vi "Throughput Test.vi"() -> ()   [LabVIEW 2017]
uses:
  logger/Logger.lvclass
panel:
  out "error IO":errorcluster
  out "tag count":i32
  out "Running":bool
  out "tag updates":i32
  out "tag publish interval":i32
  out "Iteration":i32
  in  "stop":bool
  in  "File Send Interval (Seconds)":dbl=600.0
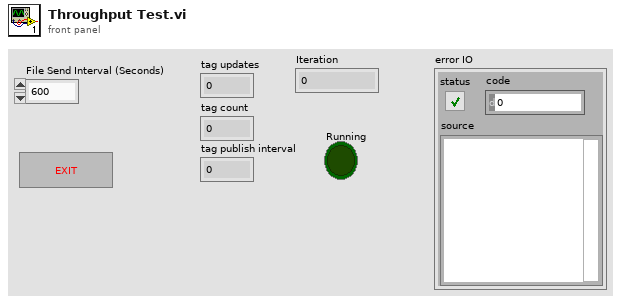
[diagram p1: front panel]
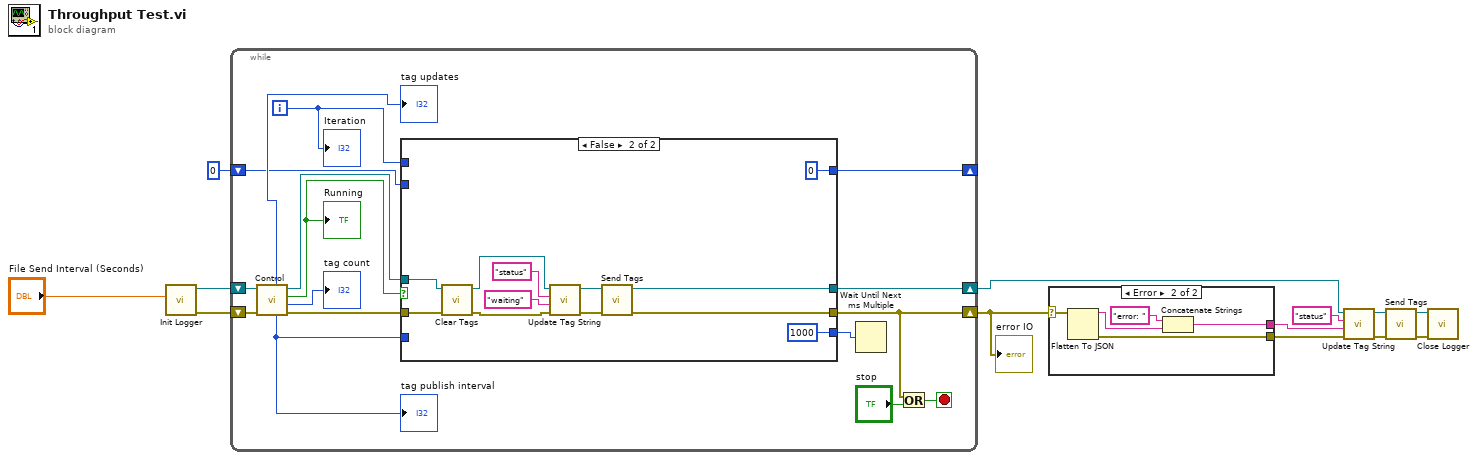
[diagram p0: block diagram]
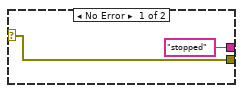
[diagram p2: hidden frame]
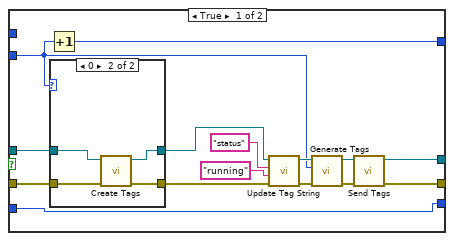
[diagram p3: hidden frame]
diagram:
  n1 = call "Init Logger.vi"("File Send Interval (Seconds)"="File Send Interval (Seconds)") -> ("error out"=w11:errorcluster, "Logger out.lvclass"=w12:refnum<class "Logger.lvclass">)  [unwired: 9 in]
  n2 = while {
    shift-right: [w24] -> w2
    shift-left: w11 -> [w19]
    shift-right: [w26] -> w6
    shift-left: w12 -> [w20]
    shift-right: [w14] -> _
    shift-left: 0 -> [w15]
    i -> [w16]
    stop <- w23 stop-if-true
    n3 = call "Control.vi"("error in (no error)"=w19, "Logger in.lvclass"=w20) -> ("error out"=w28:errorcluster, "tag count"=→"tag count":i32, "Start"=w29:bool, "Logger out.lvclass"=w27:refnum<class "Logger.lvclass">, "tag publish interval"=w18:i32, "tag updates"=→"tag updates":i32)  [unwired: 4 in]
    "tag publish interval" <- w18
    "Running" <- w29
    n4 = case shown="False" w29 {
      tunnel: w28 -> [w32 w57]
      tunnel: [w44 w62] -> w24
      tunnel: w27 -> [w30 w58]
      tunnel: [w43 w61] -> w26
      tunnel: w18 -> [w36 _]
      tunnel: [w36 1000 ("tag publish interval")] -> w17
      tunnel: w16 -> [_ _]
      tunnel: w15 -> [w34 _]
      tunnel: [w35 0] -> w14
      frame True {
        n5 = Increment(x=w34) -> (x+1=w35:i32)
        n6 = case shown="0" w34 {
          tunnel: [w46 w47] -> w33
          tunnel: w32 -> [w46 w49]
          tunnel: [w45 w48] -> w31
          tunnel: w30 -> [w45 w50]
          frame 1, Default {
          }
          frame 0 {
            n7 = call "Create Tags.vi"("error in (no error)"=w49, "Logger in.lvclass"=w50) -> ("error out"=w47:errorcluster, "Logger out.lvclass"=w48:refnum<class "Logger.lvclass">)  [unwired: 8 in]
          }
        }
        n8 = call "Update Tag String.vi"("error in (no error)"=w33, "string"="running", "Tag Path"="status", "Logger in.lvclass"=w31) -> ("error out"=w37:errorcluster, "Logger out.lvclass"=w38:refnum<class "Logger.lvclass">)  [unwired: 6 in]
        n9 = call "Generate Tags.vi"("error in (no error)"=w37, "Value"=w34, "Logger in.lvclass"=w38) -> ("error out"=w41:errorcluster, "Logger out.lvclass"=w42:refnum<class "Logger.lvclass">)  [unwired: 7 in]
        n10 = call "Send Tags.vi"("error in (no error)"=w41, "Logger in.lvclass"=w42) -> ("error out"=w44:errorcluster, "Logger out.lvclass"=w43:refnum<class "Logger.lvclass">)  [unwired: 8 in]
      }
      frame False {
        n11 = call "Clear Tags.vi"("error in (no error)"=w57, "Logger in.lvclass"=w58) -> ("error out"=w53:errorcluster, "Logger out.lvclass"=w56:refnum<class "Logger.lvclass">)  [unwired: 8 in]
        n12 = call "Update Tag String.vi"("error in (no error)"=w53, "string"="waiting", "Tag Path"="status", "Logger in.lvclass"=w56) -> ("error out"=w54:errorcluster, "Logger out.lvclass"=w55:refnum<class "Logger.lvclass">)  [unwired: 6 in]
        n13 = call "Send Tags.vi"("error in (no error)"=w54, "Logger in.lvclass"=w55) -> ("error out"=w62:errorcluster, "Logger out.lvclass"=w61:refnum<class "Logger.lvclass">)  [unwired: 8 in]
      }
    }
    n14 = Wait Until Next ms Multiple(millisecond multiple=w17) -> ()  [unwired: 1 out]
    n15 = Or(x=w24, y="stop") -> (x .or. y?=w23:bool)
    "Iteration" <- w16
  }
  "error IO" <- w2
  n16 = case shown="Error" w2 {
    selector: w2 -> [w64 w69]
    tunnel: ["stopped" ("JSON string") w65] -> w9
    tunnel: [w64 w68] -> w3
    frame No Error {
    }
    frame Error {
      n17 = Flatten To JSON(anything=w69) -> (JSON string=w66:string, 11:w68:errorcluster)  [unwired: 2 in]
      n18 = Concatenate Strings("error: " ("JSON string"), w66) -> (w65:string)
    }
  }
  n19 = call "Update Tag String.vi"("error in (no error)"=w3, "string"=w9, "Tag Path"="status", "Logger in.lvclass"=w6) -> ("error out"=w8:errorcluster, "Logger out.lvclass"=w7:refnum<class "Logger.lvclass">)  [unwired: 6 in]
  n20 = call "Send Tags.vi"("error in (no error)"=w8, "Logger in.lvclass"=w7) -> ("error out"=w5:errorcluster, "Logger out.lvclass"=w4:refnum<class "Logger.lvclass">)  [unwired: 8 in]
  n21 = call "Close Logger.vi"("error in (no error)"=w5, "Logger in.lvclass"=w4) -> ()  [unwired: 9 in, 1 out]
